vi "Size.vi"(8 "error in (no error)":errorcluster, 11 "Buffer Data in":refnum<class "Buffer.lvclass">) -> (0 "error out":errorcluster, 2 "Image Size":T1, 3 "Buffer Data":refnum<class "Buffer.lvclass">)   [LabVIEW 2020, in "Buffer.lvclass"]
uses:
  Buffer.lvclass
  Image Size.ctl
  Buffer.lvclass/Buffer.ctl
  bin/gindustrialcam_32-1.dll
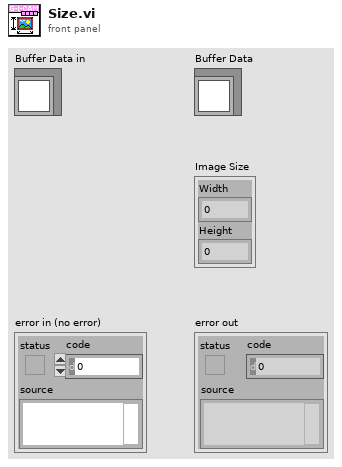
[diagram p1: front panel]
types:
  T1 = typedef "Buffer.lvclass/Image Size.ctl" = cluster{"Width":u16, "Height":u16}
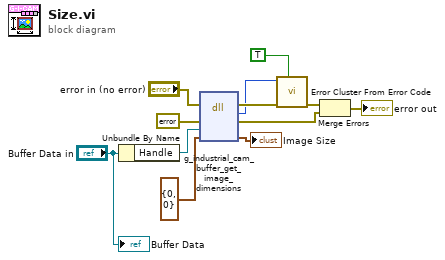
[diagram p0: block diagram]
diagram:
  n1 = Unbundle By Name("Buffer Data in") -> ("Handle"=w1:refnum<data-value>)
  n2 = dll-call lib="C:/Workspace/SSDC/g-industrial-camera/LabVIEW/g_industrial_cam/bin/gindustrialcam_*-1.*" fn="g_industrial_cam_buffer_get_image_dimensions"(error in="error in (no error)", "err"=errorcluster {"status"=FALSE, "code"=0, "source"=""} ("error constant"), "edvr"=w1, "dims"=T1 {"Width"=0, "Height"=0} ("Image Size")) -> (error out=w12:errorcluster, "Mg_Error"=w11:i32, "err"=w9:errorcluster, "dims"=→"Image Size":T1)  [unwired: 3 in, 1 out]
  n3 = call <vilib>:"Error Cluster From Error Code.vi"("show call chain? (False)"=TRUE, "error in (no error)"=w12, "error code (0)"=w11) -> ("error out"=w10:errorcluster)  [unwired: 6 in]
  n4 = Merge Errors(w10, w9) -> (→"error out":errorcluster)
  "Buffer Data" <- "Buffer Data in"
